vi "BLMPop.vi"(0 "reference in":refnum<class "Redis.lvclass">, 1 "Keys":string[](array[string]), 5 "WhereFrom":T1, 9 "Count(1)":u32=1, 11 "Error In":errorcluster, 13 "Timeout(1000ms)":i32=1000) -> (4 "reference out":refnum<class "Redis.lvclass">, 8 "Elements":string[](array[string]), 15 "Error Out":errorcluster)   [LabVIEW 2020, in "Redis.lvclass"]
doc: "<b>BLMPOP</b>\n\nBLMPOP is the blocking variant of LMPOP.\n\nWhen any of the lists contains elements, this command behaves exactly like LMPOP. When used inside a MULTI/EXEC block, this command behaves exactly like LMPOP. When all lists are empty, Redis will block the connection until another client pushes to it or until the timeout (a double value specifying the maximum number of seconds to block) elapses. A timeout of zero can be used to block indefinitely.\n\nSee LMPOP for more information.\n\nElements are popped from either the left or right of the first non-empty list based on the passed argument. The number of returned elements is limited to the lower between the non-empty list's length, and the <b>count</b> argument (which defaults to 1)."
uses:
  Redis.lvclass
  Redis.lvclass/Redis.ctl
  SideEnum.ctl
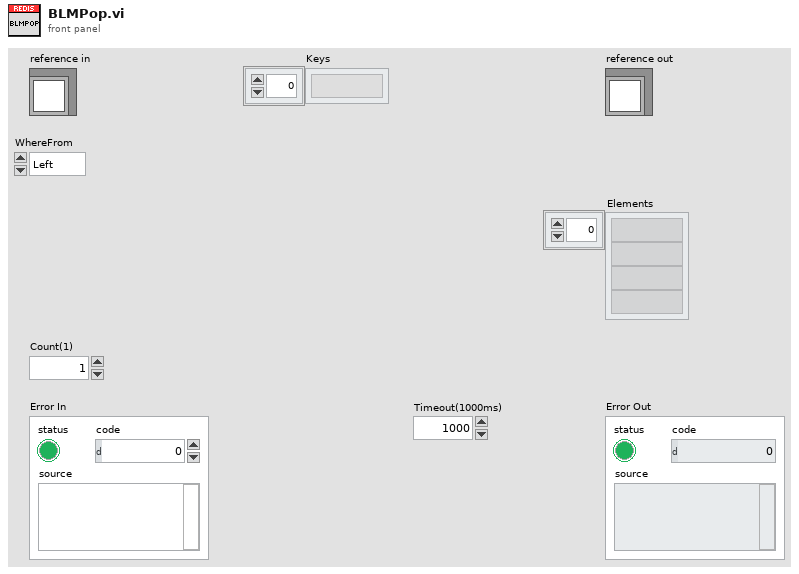
[diagram p1: front panel]
types:
  T1 = typedef "Redis.lvclass/SideEnum.ctl" = enum16{"Left", "Right"}
  T2 = typedef "Redis.lvclass/RedisDataType.ctl" = cluster{"Reply Type":T3, "Integer":i64, "String":string, "Multibulk":variant[], "StringData":string[]}
  T3 = typedef "Redis.lvclass/ReplyDataTypeEnum.ctl" = enum16{"None", "Error", "Status", "Nil", "Integer", "String", "Multibulk"}
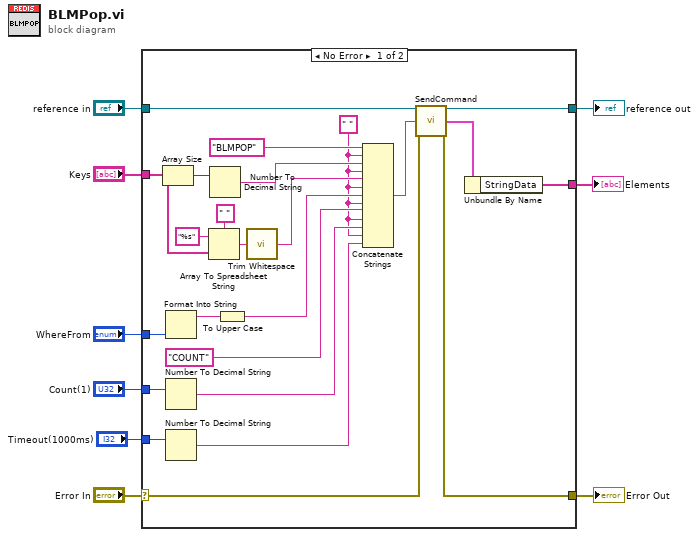
[diagram p0: block diagram]
diagram:
  n1 = case shown="No Error" "Error In" {
    selector: "Error In" -> [w31 w35]
    tunnel: [w30 w35] -> w8
    tunnel: [w33 w34] -> w6
    tunnel: "reference in" -> [w32 w34]
    tunnel: "Keys" -> [w19 _]
    tunnel: [w26 _] -> w4
    tunnel: "Count(1)" -> [w25 _]
    tunnel: "WhereFrom" -> [w21 _]
    tunnel: "Timeout(1000ms)" -> [w12 _]
    frame No Error {
      w10 = " "
      n2 = Array Size(array=w19) -> (size(s)=w24:i32)
      n3 = Format Into String(w21) -> (resulting string=w22:string)  [unwired: 3 in, 1 out]
      n4 = Number To Decimal String(number=w25) -> (decimal integer string=w14:string)  [unwired: 1 in]
      n5 = Number To Decimal String(number=w12) -> (decimal integer string=w11:string)  [unwired: 1 in]
      n6 = Array To Spreadsheet String(delimiter (Tab)=" ", array=w19, 3:"%s" ("format string")) -> (spreadsheet string=w17:string)
      n7 = Number To Decimal String(number=w24) -> (decimal integer string=w23:string)  [unwired: 1 in]
      n8 = To Upper Case(1:w22) -> (0:w16:string)
      n9 = call <vilib>:"Trim Whitespace.vi"("string"=w17) -> ("trimmed string"=w13:string)  [unwired: 1 in]
      n10 = Concatenate Strings("BLMPOP", w10, w23, w10, w13, w10, w16, w10, "COUNT", w10, w14, w10, w11) -> (w28:string)
      n11 = call "SendCommand.vi"("reference in"=w32, "Command"=w28, "Error In"=w31) -> ("reference out"=w33:refnum<class "Redis.lvclass">, "Data"=w27:T2, "Error Out"=w30:errorcluster)  [unwired: 10 in]
      n12 = Unbundle By Name(w27) -> ("StringData"=w26:string[])
    }
    frame Error {
    }
  }
  "Error Out" <- w8
  "reference out" <- w6
  "Elements" <- w4
